vi "CMN_GetPhysPath.vi"(10 "path":string) -> (2 "physical path":string)   [LabVIEW 2016]
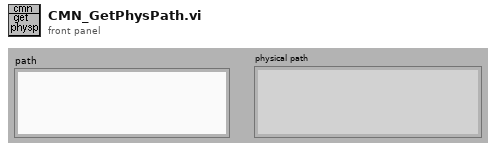
[diagram p1: front panel]
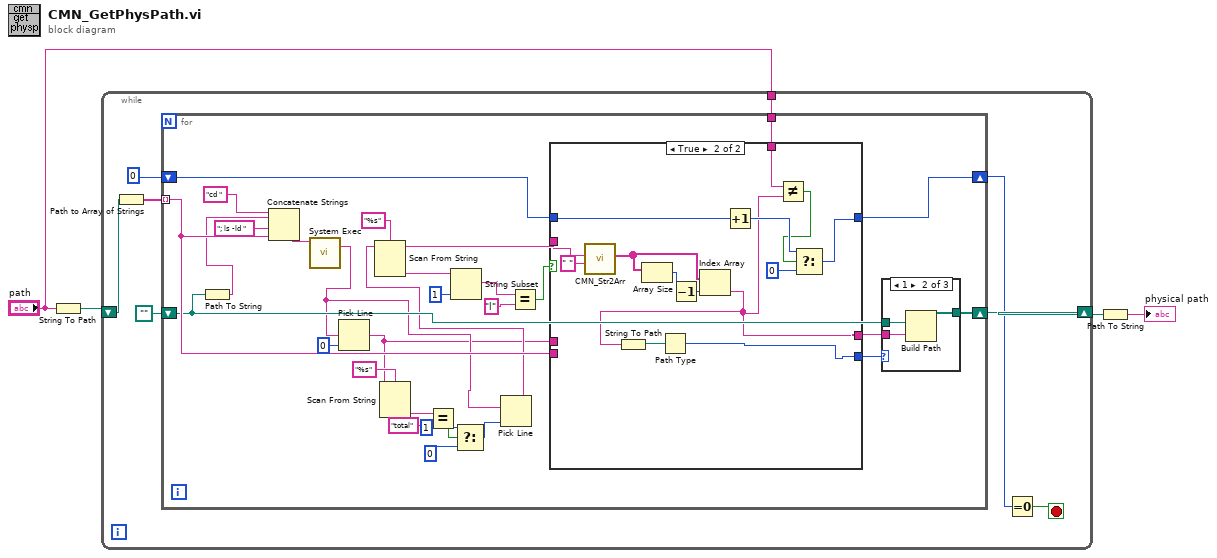
[diagram p0: block diagram]
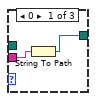
[diagram p2: hidden frame]
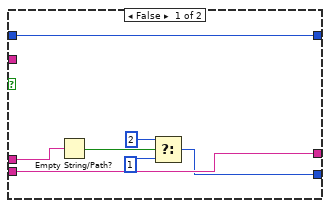
[diagram p4: hidden frame]
diagram:
  n1 = String To Path(string="path") -> (path=w3:path)
  n2 = while {
    shift-right: [w9] -> w4
    shift-left: w3 -> [w6]
    tunnel: "path" -> [w5]
    stop <- w7 stop-if-true
    n3 = Path to Array of Strings(0:w6) -> (2:w12:string[])  [unwired: 1 out]
    n4 = for {
      tunnel: w12 -> [w33] mode=indexing
      shift-right: [w35] -> w9
      shift-left: path "" ("appended path") -> [w32]
      shift-right: [w28] -> w8
      shift-left: 0 -> [w29]
      tunnel: w5 -> [w13]
      n5 = Path To String(path=w32) -> (string=w30:string)
      n6 = Concatenate Strings("cd " ("string"), w30, "; ls -ld " ("string"), w33) -> (w42:string)
      n7 = call <vilib>:"System Exec.vi"("command line"=w42) -> ("standard output"=w23:string)  [unwired: 5 in, 5 out]
      n8 = Pick Line(multi-line string=w23, line index=0) -> (output string=w16:string)  [unwired: 1 out]
      n9 = Scan From String(format string="%s", input string=w16) -> (output 1=w25:string)  [unwired: 2 in, 4 out]
      n10 = Equal?(x=w25, y="total") -> (x = y?=w22:bool)
      n11 = Select(t=1, s=w22, f=0 ("line index")) -> (s? t:f=w19:i32)
      n12 = Pick Line(multi-line string=w23, line index=w19) -> (output string=w18:string)  [unwired: 1 out]
      n13 = Scan From String(format string="%s", input string=w18) -> (remaining string=w15:string, output 1=w40:string)  [unwired: 2 in, 3 out]
      n14 = String Subset(string=w40, length (rest)=1 ("length (rest)")) -> (substring=w37:string)  [unwired: 1 out]
      n15 = Equal?(x=w37, y="l") -> (x = y?=w14:bool)
      n16 = case shown="True" w14 {
        tunnel: w15 -> [_ w68]
        tunnel: [w55 w58] -> w34
        tunnel: w33 -> [w55 _]
        tunnel: w29 -> [w54 w69]
        tunnel: [w54 w61] -> w28
        tunnel: [w50 w56] -> w17
        tunnel: w16 -> [w53 _]
        tunnel: w13 -> [_ w59]
        frame False {
          n17 = Empty String/Path?(string/path=w53) -> (empty?=w52:bool)
          n18 = Select(t=i16 2, s=w52, f=i16 1 ("type")) -> (s? t:f=w50:i16)
        }
        frame True {
          n19 = call "CMN_Str2Arr.vi"("separator"=" ", "string in"=w68) -> ("Array out"=w66:string[])  [unwired: 2 in, 7 out]
          n20 = Array Size(array=w66) -> (size(s)=w65:i32)
          n21 = Decrement(x=w65) -> (x-1=w64:i32)
          n22 = Index Array(array=w66, index=w64) -> (element=w58:string)
          n23 = String To Path(string=w58) -> (path=w63:path)
          n24 = Path Type(1:w63) -> (0:w56:i16)
          n25 = Increment(x=w69) -> (x+1=w62:i32)
          n26 = Not Equal?(x=w59, y=w58) -> (x != y?=w57:bool)
          n27 = Select(t=w62, s=w57, f=0) -> (s? t:f=w61:i32)
        }
      }
      n28 = case shown="1" w17 {
        tunnel: [w43 w47 w48] -> w35
        tunnel: w34 -> [w44 w46 _]
        tunnel: w32 -> [_ w45 w48]
        frame 0 {
          n29 = String To Path(string=w44) -> (path=w43:path)
        }
        frame 1 {
          n30 = Build Path(base path=w45, name or relative path=w46) -> (appended path=w47:path)
        }
        frame Default {
        }
      }
    }
    n31 = Equal To 0?(x=w8) -> (x = 0?=w7:bool)
  }
  n32 = Path To String(path=w4) -> (string=→"physical path":string)
